vi "stopwatch.vi"() -> ()   [LabVIEW 2023]
panel:
  in  "stop":bool
  out "ms":dbl format="%0#3.0f"
  out "Seconds":dbl format="%0#2.0f"
  out "Minutes":dbl format="%0#2.1f"
  out "Hours":dbl format="%0#2.1f"
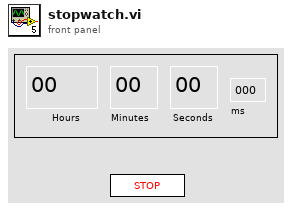
[diagram p1: front panel]
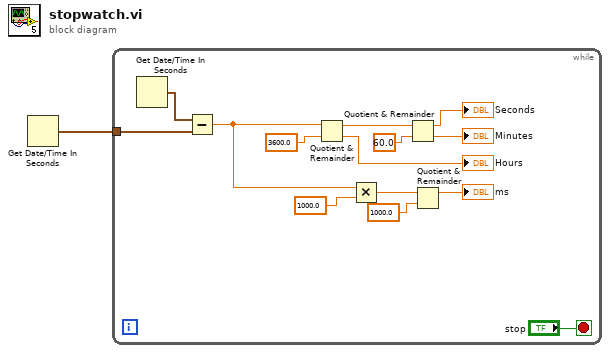
[diagram p0: block diagram]
diagram:
  n1 = Get Date/Time In Seconds() -> (seconds since 1Jan1904=w1:timestamp)
  n2 = while {
    tunnel: w1 -> [w14]
    stop <- "stop" stop-if-true
    n3 = Get Date/Time In Seconds() -> (seconds since 1Jan1904=w13:timestamp)
    n4 = Subtract(x=w13, y=w14) -> (x-y=w6:dbl)
    n5 = Quotient & Remainder(x=w6, y=3600.0) -> (x-y*floor(x/y)=w10:dbl, floor(x/y)=→"Hours":dbl)
    n6 = Multiply(x=w6, y=1000.0) -> (x*y=w4:dbl)
    n7 = Quotient & Remainder(x=w10, y=60.0) -> (x-y*floor(x/y)=→"Seconds":dbl, floor(x/y)=→"Minutes":dbl)
    n8 = Quotient & Remainder(x=w4, y=1000.0) -> (x-y*floor(x/y)=→"ms":dbl)  [unwired: 1 out]
  }
